vi "YOLOTrack-1.0.vi"() -> ()   [LabVIEW 2016]
uses:
  <vilib>/vision/NI_Vision_Development_Module.lvlib
panel:
  out "Status":string
  out "Device Name":string
  out "setupYOLO Return":i32
  out "Model Imported":bool
  out "GPU Support":bool
  out "Init.":bool
  out "Path to YOLO DLL":path
  out "Class Colors":u32[](array[colorbox])=[65535, 16776960, 16711680, 6618880, 255]
  out "Input Tensor":sgl[][][](array[numeric])
  out "Output Size":i32
  out "Output Tensor":sgl[](array[numeric])
  out "Input Size":i32
  out "setupTF Return":i32
  out "Input Shape":i64[](array[numeric])
  out "Output Shape":i64[](array[numeric])
  out "IMAGE_H":i32
  out "IMAGE_W":i32
  out "GRID_H":i32
  out "GRID_W":i32
  out "BOXES":i32
  out "CLASSES":i32
  out "ANCHORS":sgl[](array[numeric]) format="%.2g"
  out "INPUT_NODE_NAME":string
  out "OUTPUT_NODE_NAME":string
  out "TensorFlow Version":string
  out "Path to TF DLL":path
  out "N_MAX":i32=100
  in  "NMS Threshold":sgl(slide)=0.45 min=0 max=1 step=0.01 scale=0.0..1.0
  in  "Obj. Threshold":sgl(slide)=0.5 min=0 max=1 step=0.01 scale=0.0..1.0
  out "TensorFlow":bool
  out "Run:":dbl format="%.2f"
  out "runTF Return":i32
  in  "Path to Model":path
  out "Classes":i32[](array[numeric])
  out "N":i32
  out "decodeYOLO Return":i32
  out "X Centers":sgl[](array[numeric]) format="%.3g"
  out "Y Centers":sgl[](array[numeric]) format="%.3g"
  out "Widths":sgl[](array[numeric]) format="%.3g"
  out "Heights":sgl[](array[numeric]) format="%.3g"
  out "Decode:":dbl format="%.2f"
  in  "Path to Image":path
  out "Input Image":T1(plugin-control)
  in  "Update":bool
  in  "Stop":bool
  # "Debug Information"
  # "Timings [ms]:"
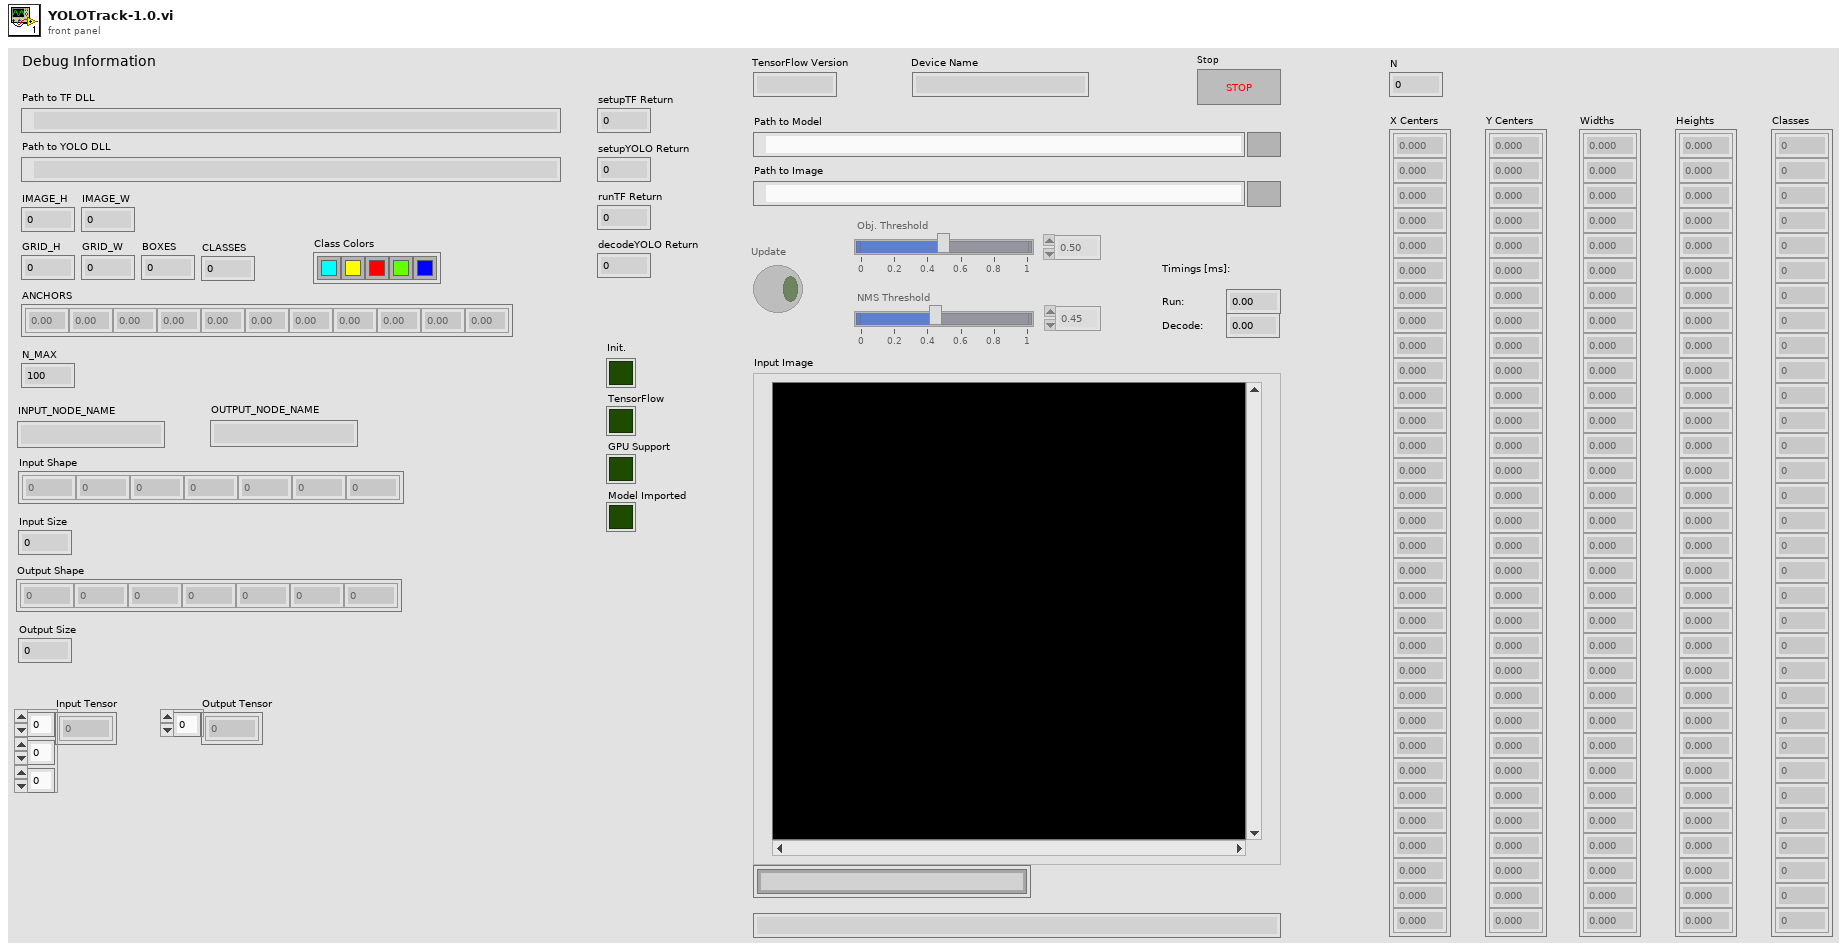
[diagram p1: front panel]
types:
  T1 = typedef "IMAQ Image.ctl" = refnum<image>
  T2 = enum8{"Enabled", "Disabled", "Disabled and Grayed Out"}
  T3 = typedef "Image Type" = u32
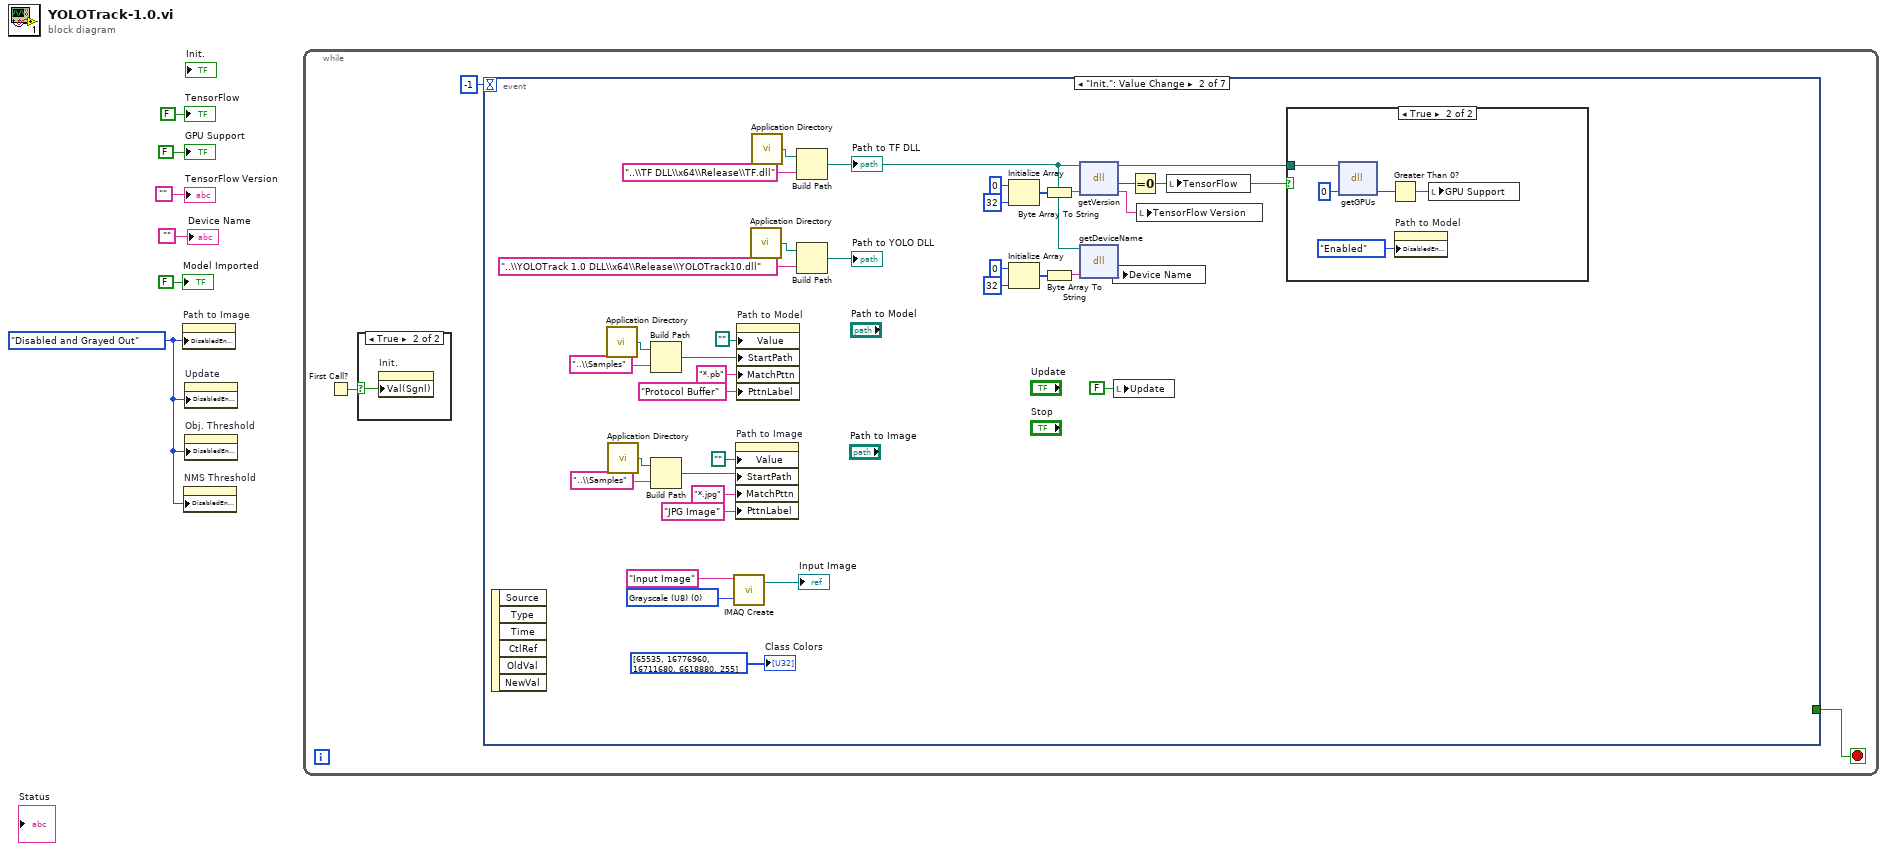
[diagram p0: block diagram]
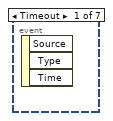
[diagram p2: hidden frame]
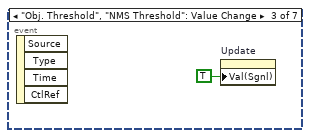
[diagram p4: hidden frame]
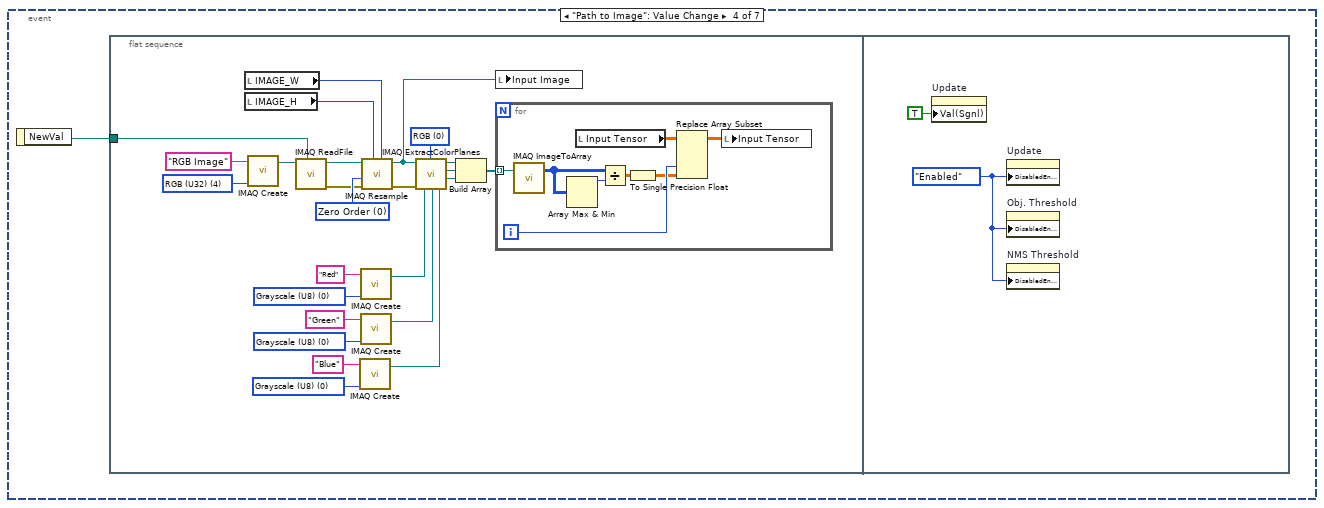
[diagram p5: hidden frame]
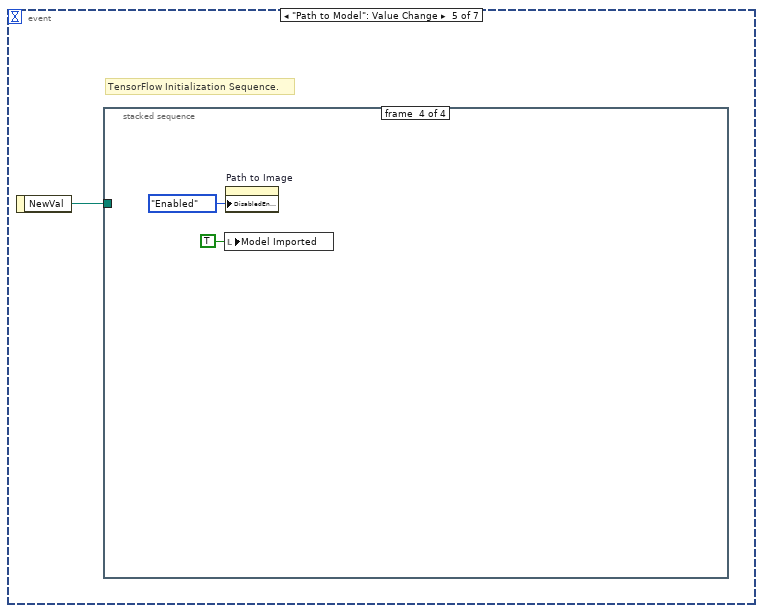
[diagram p6: hidden frame]
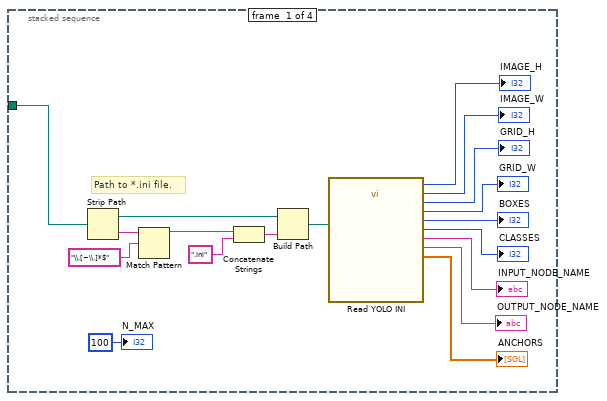
[diagram p7: hidden frame]
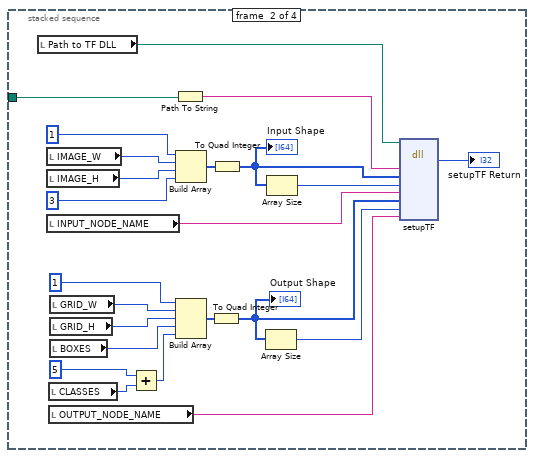
[diagram p8: hidden frame]
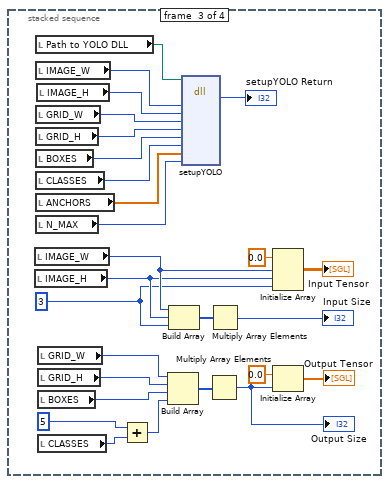
[diagram p9: hidden frame]
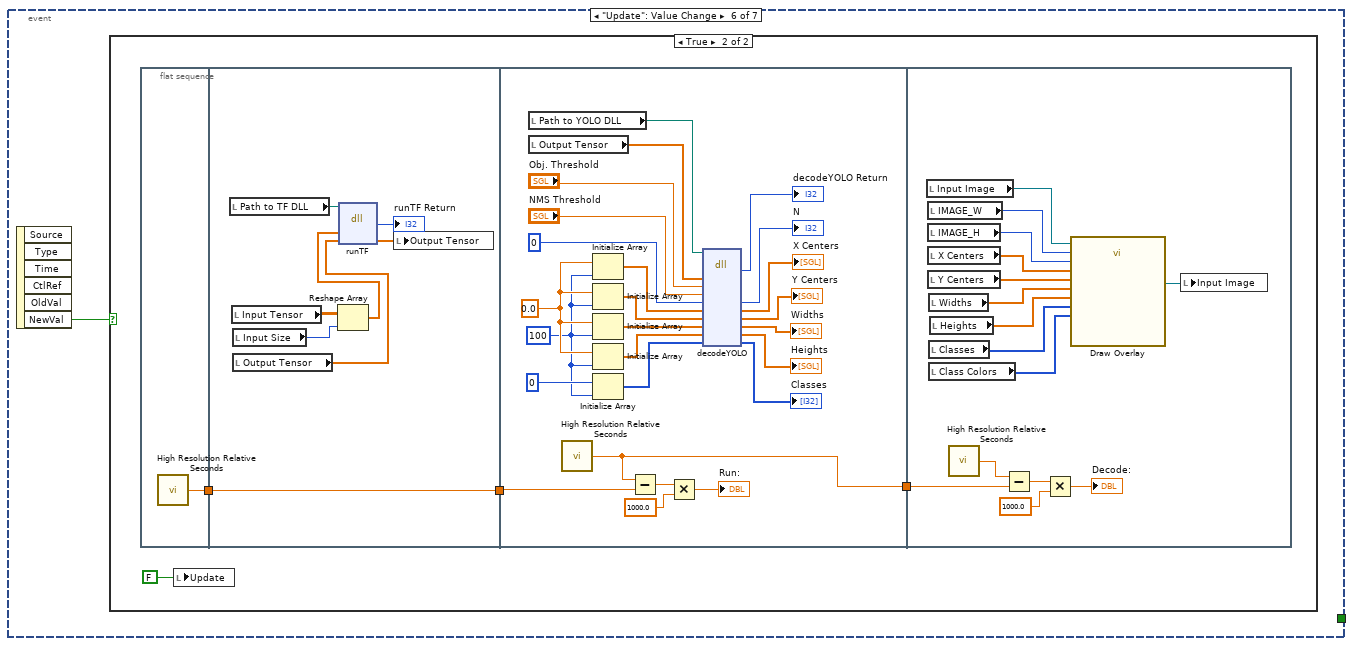
[diagram p10: hidden frame]
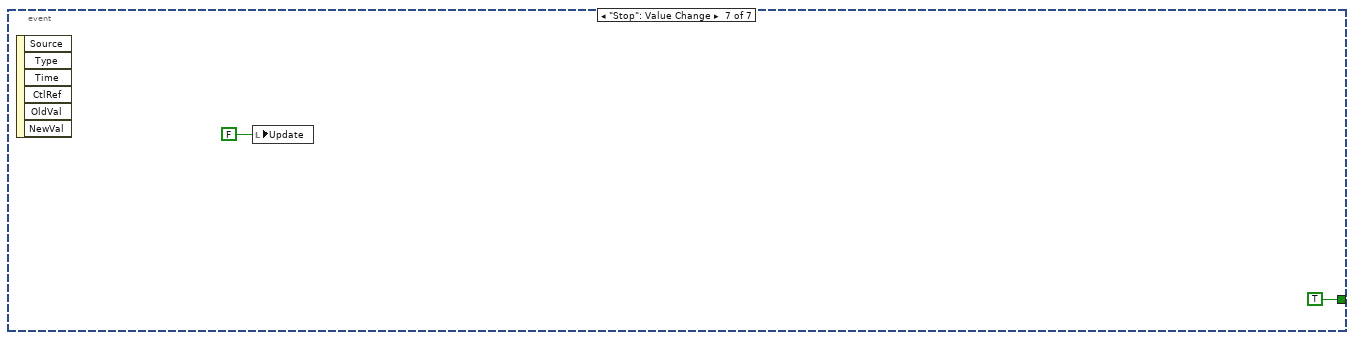
[diagram p12: hidden frame]
diagram:
  w2 = T2."Disabled and Grayed Out" ("Disabled")
  n1 = property on="Path to Image" class="Path"("DisabledEnum"=w2) -> ()  [unwired: 2 in, 2 out]
  n2 = property on="NMS Threshold" class="Slide (strict)"("DisabledEnum"=w2) -> ()  [unwired: 2 in, 2 out]
  n3 = property on="Update" class="Bool (strict)"("DisabledEnum"=w2) -> ()  [unwired: 2 in, 2 out]
  n4 = property on="Obj. Threshold" class="Slide (strict)"("DisabledEnum"=w2) -> ()  [unwired: 2 in, 2 out]
  n5 = while {
    stop <- w9 stop-if-true
    n6 = First Call?() -> (First Call?: T/F=w8:bool)
    n7 = case shown="True" w8 {
      selector: w8 -> [_ w215]
      frame False {
      }
      frame True {
        n8 = property on="Init." class="Bool (strict)"("Val(Sgnl)"=w215) -> ()  [unwired: 2 in, 2 out]
      }
    }
    n9 = event shown="[1] \"Init.\": Value Change" {
      selector: _ -> [_ _ _ _ _ _ _]
      dyn-events: _ -> [_ _ _ _ _ _ _]
      timeout: -1 -> [_ _ _ _ _ _ _]
      tunnel: [_ _ _ _ _ _ TRUE] -> w9
      event Timeout {
        n10 = event-data() -> ()  [unwired: 1 in, 3 out]
      }
      event "Init.": Value Change {
        w34 = T3 0 items=["Grayscale (U8)", "Grayscale (I16)", "Grayscale (SGL)", "Complex (CSG)", "RGB (U32)", "HSL (U32)", "RGB (U64)", "Grayscale (U16)"] ("Image Type")
        n11 = event-data() -> ()  [unwired: 1 in, 6 out]
        n12 = call <vilib>:"Application Directory.vi"() -> ("Application Directory"=w38:path)
        n13 = call <vilib>:"Application Directory.vi"() -> ("Application Directory"=w42:path)
        n14 = Build Path(base path=w38, name or relative path="..\\Samples" ("string")) -> (appended path=w45:path)
        n15 = Build Path(base path=w42, name or relative path="..\\Samples" ("string")) -> (appended path=w41:path)
        n16 = call "IMAQ Create"("Image Name"="Input Image", "Image Type"=w34) -> ("New Image"=→"Input Image":T1)  [unwired: 3 in, 1 out]
        n17 = property on="Path to Image" class="Path"("Value"=path "", "StartPath"=w41, "MatchPttn"="*.jpg" ("string"), "PttnLabel"="JPG Image" ("string")) -> ()  [unwired: 2 in, 2 out]
        n18 = property on="Path to Model" class="Path"("Value"=path "", "StartPath"=w45, "MatchPttn"="*.pb" ("string"), "PttnLabel"="Protocol Buffer" ("string")) -> ()  [unwired: 2 in, 2 out]
        n19 = call <vilib>:"Application Directory.vi"() -> ("Application Directory"=w27:path)
        n20 = call <vilib>:"Application Directory.vi"() -> ("Application Directory"=w33:path)
        n21 = Build Path(base path=w33, name or relative path="..\\TF DLL\\x64\\Release\\TF.dll" ("string")) -> (appended path=w10:path)
        "Path to TF DLL" <- w10
        n22 = Build Path(base path=w27, name or relative path="..\\YOLOTrack 1.0 DLL\\x64\\Release\\YOLOTrack10.dll" ("string")) -> (appended path=→"Path to YOLO DLL":path)
        n23 = Initialize Array(u8 0 ("dimension size"), 32 ("dimension size")) -> (w20:u8[])
        n24 = Initialize Array(u8 0 ("dimension size"), 32 ("dimension size")) -> (w14:u8[])
        n25 = Byte Array To String(unsigned byte array=w20) -> (string=w22:string)
        n26 = Byte Array To String(unsigned byte array=w14) -> (string=w12:string)
        n27 = dll-call lib="?" fn="getVersion"(path in=w10, "tf_version"=w22) -> (path out=w18:path, "return type"=w19:i32, "tf_version"=w16:string)  [unwired: 2 in, 1 out]
        n28 = dll-call lib="?" fn="getDeviceName"(path in=w10, "gpu_name"=w12) -> ("gpu_name"=w15:string)  [unwired: 3 in, 2 out]
        n29 = local write "Device Name"(w15) -> ()
        n30 = local write "Update"(FALSE ("Update")) -> ()
        n31 = Equal To 0?(x=w19) -> (x = 0?=w17:bool)
        n32 = local write "TensorFlow Version"(w16) -> ()
        n33 = local write "TensorFlow"(w17) -> ()
        n34 = case shown="True" w17 {
          tunnel: w18 -> [_ w50]
          frame False {
          }
          frame True {
            n35 = dll-call lib="?" fn="getGPUs"(path in=w50, "int"=0) -> ("int"=w46:i32)  [unwired: 3 in, 2 out]
            n36 = Greater Than 0?(x=w46) -> (x > 0?=w49:bool)
            n37 = property on="Path to Model" class="Path"("DisabledEnum"=T2."Enabled" ("Disabled")) -> ()  [unwired: 2 in, 2 out]
            n38 = local write "GPU Support"(w49) -> ()
          }
        }
        "Class Colors" <- u32[] [65535, 16776960, 16711680, 6618880, 255]
      }
      event "Obj. Threshold", "NMS Threshold": Value Change {
        n39 = event-data() -> ()  [unwired: 1 in, 4 out]
        n40 = property on="Update" class="Bool (strict)"("Val(Sgnl)"=TRUE ("Value (Signaling)")) -> ()  [unwired: 2 in, 2 out]
      }
      event "Path to Image": Value Change {
        n41 = event-data() -> ("NewVal"=w52:path)  [unwired: 1 in]
        n42 = flat-sequence {
          tunnel: w52 -> [w61]
          frame #0 {
            w68 = T3 0 items=["Grayscale (U8)", "Grayscale (I16)", "Grayscale (SGL)", "Complex (CSG)", "RGB (U32)", "HSL (U32)", "RGB (U64)", "Grayscale (U16)"] ("Image Type")
            w67 = T3 0 items=["Grayscale (U8)", "Grayscale (I16)", "Grayscale (SGL)", "Complex (CSG)", "RGB (U32)", "HSL (U32)", "RGB (U64)", "Grayscale (U16)"] ("Image Type")
            w64 = T3 0 items=["Grayscale (U8)", "Grayscale (I16)", "Grayscale (SGL)", "Complex (CSG)", "RGB (U32)", "HSL (U32)", "RGB (U64)", "Grayscale (U16)"] ("Image Type")
            w63 = u16 0 items=["RGB", "HSL", "HSV", "HSI"] ("Color Mode")
            w73 = T3 4 items=["Grayscale (U8)", "Grayscale (I16)", "Grayscale (SGL)", "Complex (CSG)", "RGB (U32)", "HSL (U32)", "RGB (U64)", "Grayscale (U16)"] ("Image Type")
            w76 = u32 0 items=["Zero Order", "Bi-Linear", "Quadratic", "Cubic Spline"] ("Interpolation Type")
            n43 = local read "IMAGE_W"() -> (w58:i32)
            n44 = local read "IMAGE_H"() -> (w59:i32)
            n45 = call "IMAQ Create"("Image Name"="RGB Image", "Image Type"=w73) -> ("New Image"=w60:T1)  [unwired: 3 in, 1 out]
            n46 = call "IMAQ ReadFile"("File Path"=w61, "Image"=w60) -> ("error out"=w75:errorcluster, "Image Out"=w77:T1)  [unwired: 5 in, 3 out]
            n47 = call "IMAQ Create"("Image Name"="Blue", "Image Type"=w68) -> ("New Image"=w72:T1)  [unwired: 3 in, 1 out]
            n48 = call "IMAQ Create"("Image Name"="Red", "Image Type"=w64) -> ("New Image"=w70:T1)  [unwired: 3 in, 1 out]
            n49 = call "IMAQ Create"("Image Name"="Green", "Image Type"=w67) -> ("New Image"=w71:T1)  [unwired: 3 in, 1 out]
            n50 = call "IMAQ Resample"("X Resolution"=w58, "Y Resolution"=w59, "error in (no error)"=w75, "Interpolation Type"=w76, "Image Src"=w77) -> ("error out"=w62:errorcluster, "Image Dst Out"=w53:T1)  [unwired: 5 in]
            n51 = call "IMAQ ExtractColorPlanes"("Blue or Luma or Val or Inten Plane"=w72, "Color Mode"=w63, "error in (no error)"=w62, "Green or Sat Plane"=w71, "Red or Hue Plane"=w70, "Image Src"=w53) -> ("Blue or Luma or Val or Inten Plane out"=w54:T1, "Green or Sat Plane out"=w55:T1, "Red or Hue Plane out"=w56:T1)  [unwired: 2 in, 1 out]
            n52 = Build Array(w56, w55, w54) -> (w57:T1[])
            n53 = local write "Input Image"(w53) -> ()
            n54 = for {
              tunnel: w57 -> [w85] mode=indexing
              i -> [w80]
              n55 = call "IMAQ ImageToArray"("Image"=w85) -> ("Image Pixels (U8)"=w84:u8[][])  [unwired: 3 in, 4 out]
              n56 = Array Max & Min(array=w84) -> (max value=w83:u8)  [unwired: 3 out]
              n57 = local read "Input Tensor"() -> (w82:sgl[][][])
              n58 = Divide(x=w84, y=w83) -> (x/y=w79:dbl[][])
              n59 = To Single Precision Float(number=w79) -> (single precision float=w78:sgl[][])
              n60 = Replace Array Subset(array=w82, new element=w78, index (dim 2)=w80) -> (w81:sgl[][][])  [unwired: 2 in]
              n61 = local write "Input Tensor"(w81) -> ()
            }
          }
          frame #1 {
            w86 = T2."Enabled" ("Disabled")
            n62 = property on="Update" class="Bool (strict)"("Val(Sgnl)"=TRUE ("Value (Signaling)")) -> ()  [unwired: 2 in, 2 out]
            n63 = property on="Update" class="Bool (strict)"("DisabledEnum"=w86) -> ()  [unwired: 2 in, 2 out]
            n64 = property on="Obj. Threshold" class="Slide (strict)"("DisabledEnum"=w86) -> ()  [unwired: 2 in, 2 out]
            n65 = property on="NMS Threshold" class="Slide (strict)"("DisabledEnum"=w86) -> ()  [unwired: 2 in, 2 out]
          }
        }
      }
      event "Path to Model": Value Change {
        # "TensorFlow Initialization Sequence."
        n66 = event-data() -> ("NewVal"=w88:path)  [unwired: 1 in]
        n67 = stacked-sequence {
          tunnel: w88 -> [w89 w107 _ _]
          frame #0 {
            # "Path to *.ini file."
            n68 = Strip Path(path=w89) -> (stripped path=w96:path, name=w95:string)
            n69 = Match Pattern(string=w95, regular expression="\\.[~\\.]*$") -> (before substring=w93:string)  [unwired: 4 out]
            n70 = Concatenate Strings(w93, ".ini" ("string")) -> (w92:string)
            n71 = Build Path(base path=w96, name or relative path=w92) -> (appended path=w90:path)
            n72 = call "Read YOLO INI.vi"("Path to INI"=w90) -> ("OUTPUT_NAME"=→"OUTPUT_NODE_NAME":string, "ANCHORS"=→"ANCHORS":sgl[], "INPUT_NAME"=→"INPUT_NODE_NAME":string, "IMAGE_H"=→"IMAGE_H":i32, "IMAGE_W"=→"IMAGE_W":i32, "GRID_H"=→"GRID_H":i32, "GRID_W"=→"GRID_W":i32, "BOXES"=→"BOXES":i32, "CLASSES"=→"CLASSES":i32)  [unwired: 10 in]
            "N_MAX" <- 100 ("N_MAX")
          }
          frame #1 {
            n73 = local read "Path to TF DLL"() -> (w109:path)
            n74 = local read "IMAGE_W"() -> (w120:i32)
            n75 = local read "IMAGE_H"() -> (w121:i32)
            n76 = local read "INPUT_NODE_NAME"() -> (w111:string)
            n77 = local read "CLASSES"() -> (w115:i32)
            n78 = local read "OUTPUT_NODE_NAME"() -> (w114:string)
            n79 = local read "GRID_W"() -> (w118:i32)
            n80 = local read "GRID_H"() -> (w117:i32)
            n81 = local read "BOXES"() -> (w116:i32)
            n82 = Add(x=5, y=w115) -> (x+y=w127:i32)
            n83 = Path To String(path=w107) -> (string=w129:string)
            n84 = Build Array(1 ("element"), w120, w121, 3 ("element")) -> (w124:i32[])
            n85 = Build Array(1 ("element"), w118, w117, w116, w127) -> (w125:i32[])
            n86 = To Quad Integer(1:w125) -> (0:w110:i64[])
            "Output Shape" <- w110
            n87 = To Quad Integer(1:w124) -> (0:w119:i64[])
            "Input Shape" <- w119
            n88 = Array Size(array=w110) -> (size(s)=w113:i32)
            n89 = Array Size(array=w119) -> (size(s)=w112:i32)
            n90 = dll-call lib="?" fn="setupTF"(path in=w109, "file"=w129, "in_shape"=w119, "in_dim"=w112, "in_name"=w111, "out_shape"=w110, "out_dim"=w113, "out_name"=w114) -> ("return type"=→"setupTF Return":i32)  [unwired: 9 in, 2 out]
          }
          frame #2 {
            w132 = 3 ("dimension size")
            n91 = local read "IMAGE_W"() -> (w134:i32)
            n92 = local read "IMAGE_H"() -> (w133:i32)
            n93 = local read "Path to YOLO DLL"() -> (w149:path)
            n94 = local read "IMAGE_W"() -> (w156:i32)
            n95 = local read "GRID_W"() -> (w154:i32)
            n96 = local read "GRID_H"() -> (w153:i32)
            n97 = local read "BOXES"() -> (w152:i32)
            n98 = local read "CLASSES"() -> (w151:i32)
            n99 = local read "ANCHORS"() -> (w150:sgl[])
            n100 = local read "N_MAX"() -> (w131:i32)
            n101 = local read "IMAGE_H"() -> (w155:i32)
            n102 = local read "GRID_W"() -> (w146:i32)
            n103 = local read "GRID_H"() -> (w145:i32)
            n104 = local read "BOXES"() -> (w144:i32)
            n105 = local read "CLASSES"() -> (w142:i32)
            n106 = Add(x=5 ("dimension size"), y=w142) -> (x+y=w141:i32)
            n107 = Build Array(w146, w145, w144, w141) -> (w139:i32[])
            n108 = Build Array(w134, w133, w132) -> (w136:i32[])
            n109 = dll-call lib="?" fn="setupYOLO"(path in=w149, "image_w"=w156, "image_h"=w155, "grid_w"=w154, "grid_h"=w153, "boxes"=w152, "classes"=w151, "anchors"=w150, "n"=w131) -> ("return type"=→"setupYOLO Return":i32)  [unwired: 10 in, 2 out]
            n110 = Multiply Array Elements(1:w139) -> (0:w138:i32)
            "Output Size" <- w138
            n111 = Multiply Array Elements(1:w136) -> (0:→"Input Size":i32)
            n112 = Initialize Array(sgl 0.0, w134, w133, w132) -> (→"Input Tensor":sgl[][][])
            n113 = Initialize Array(sgl 0.0 ("element"), w138) -> (→"Output Tensor":sgl[])
          }
          frame #3 {
            n114 = local write "Model Imported"(TRUE ("Model Imported")) -> ()
            n115 = property on="Path to Image" class="Path"("DisabledEnum"=T2."Enabled" ("Disabled")) -> ()  [unwired: 2 in, 2 out]
          }
        }
      }
      event "Update": Value Change {
        n116 = event-data() -> ("NewVal"=w159:bool)  [unwired: 1 in, 5 out]
        n117 = case shown="True" w159 {
          frame False {
          }
          frame True {
            n118 = flat-sequence {
              tunnel: [w164] -> w161
              tunnel: [w171] -> w162
              tunnel: w161 -> [w171]
              tunnel: w162 -> [w181]
              tunnel: [w180] -> w160
              tunnel: w160 -> [w208]
              frame #0 {
                n119 = call <vilib>:"High Resolution Relative Seconds.vi"() -> ("relative seconds"=w164:dbl)
              }
              frame #1 {
                n120 = local read "Path to TF DLL"() -> (w169:path)
                n121 = local read "Input Tensor"() -> (w172:sgl[][][])
                n122 = local read "Input Size"() -> (w170:i32)
                n123 = local read "Output Tensor"() -> (w166:sgl[])
                n124 = Reshape Array(w172, w170) -> (w167:sgl[])
                n125 = dll-call lib="?" fn="runTF"(path in=w169, "input_tensor"=w167, "output_tensor"=w166) -> ("return type"=→"runTF Return":i32, "output_tensor"=w165:sgl[])  [unwired: 3 in, 2 out]
                n126 = local write "Output Tensor"(w165) -> ()
              }
              frame #2 {
                w178 = 100 ("dimension size")
                w179 = sgl 0.0 ("element")
                n127 = local read "Path to YOLO DLL"() -> (w196:path)
                n128 = local read "Output Tensor"() -> (w173:sgl[])
                n129 = call <vilib>:"High Resolution Relative Seconds.vi"() -> ("relative seconds"=w180:dbl)
                n130 = Initialize Array(w179, w178) -> (w194:sgl[])
                n131 = Initialize Array(w179, w178) -> (w193:sgl[])
                n132 = Initialize Array(w179, w178) -> (w192:sgl[])
                n133 = Initialize Array(w179, w178) -> (w197:sgl[])
                n134 = Initialize Array(0, w178) -> (w187:i32[])
                n135 = Subtract(x=w180, y=w181) -> (x-y=w184:dbl)
                n136 = Multiply(x=w184, y=1000.0) -> (x*y=→"Run:":dbl)
                n137 = dll-call lib="?" fn="decodeYOLO"(path in=w196, "output_tensor"=w173, "obj_threshold"="Obj. Threshold", "nms_threshold"="NMS Threshold", "n_out"=0, "x_out"=w194, "y_out"=w193, "w_out"=w192, "h_out"=w197, "c_cout"=w187) -> ("return type"=→"decodeYOLO Return":i32, "n_out"=→"N":i32, "x_out"=→"X Centers":sgl[], "y_out"=→"Y Centers":sgl[], "w_out"=→"Widths":sgl[], "h_out"=→"Heights":sgl[], "c_cout"=→"Classes":i32[])  [unwired: 5 in, 2 out]
              }
              frame #3 {
                n138 = local read "Input Image"() -> (w200:T1)
                n139 = local read "IMAGE_W"() -> (w199:i32)
                n140 = local read "IMAGE_H"() -> (w198:i32)
                n141 = local read "X Centers"() -> (w206:sgl[])
                n142 = local read "Y Centers"() -> (w205:sgl[])
                n143 = local read "Widths"() -> (w204:sgl[])
                n144 = local read "Classes"() -> (w202:i32[])
                n145 = local read "Class Colors"() -> (w201:u32[])
                n146 = local read "Heights"() -> (w203:sgl[])
                n147 = call <vilib>:"High Resolution Relative Seconds.vi"() -> ("relative seconds"=w212:dbl)
                n148 = Subtract(x=w212, y=w208) -> (x-y=w211:dbl)
                n149 = Multiply(x=w211, y=1000.0) -> (x*y=→"Decode:":dbl)
                n150 = call "Draw Overlay.vi"("Image (in)"=w200, "Image Width (in)"=w199, "Image Height (in)"=w198, "X Center (in)"=w206, "Y Center (in)"=w205, "Height (in)"=w204, "Colors (in)"=w201, "Width (in)"=w203, "Classes (in)"=w202) -> ("Image (out)"=w207:T1)  [unwired: 10 in]
                n151 = local write "Input Image"(w207) -> ()
              }
            }
            n152 = local write "Update"(FALSE ("Update SLM")) -> ()
          }
        }
      }
      event "Stop": Value Change {
        n153 = event-data() -> ()  [unwired: 1 in, 6 out]
        n154 = local write "Update"(FALSE ("Update SLM")) -> ()
      }
    }
  }
  "TensorFlow" <- FALSE ("TensorFlow")
  "GPU Support" <- FALSE ("TensorFlow")
  "TensorFlow Version" <- ""
  "Model Imported" <- FALSE ("Model Import")
  "Device Name" <- ""
